vi "Write Pulse Recorder Configuration.vi"(8 "error in (no error)":errorcluster, 10 "Configuration":T1={"Pre-trigger duration"=0.01, "Post-trigger duration"=0.1, "Rate"=1000000.0, "Ranges"=[10.0], "Re-name channels"=[], "Active channels"="0:1", "External clock"=FALSE} {"Rate" format="%#_8pHz"; "Post-trigger duration" format="%#_6ps"; "Pre-trigger duration" format="%#_6ps"; "Ranges" format="%#_6pV"}, 11 "RP Delayed in":refnum<class "RP Level.lvclass">) -> (0 "error out":errorcluster, 3 "RP Delayed out":refnum<class "RP Level.lvclass">)   [LabVIEW 2016, in "RP Level.lvclass"]
uses:
  RP Level.lvclass
  NHMFL_Core/Libraries/Instruments/Pulse Driver/Pusle Driver Configuration.ctl
  NHMFL_Core/Libraries/Red Pitaya/RP Level Configuration.ctl
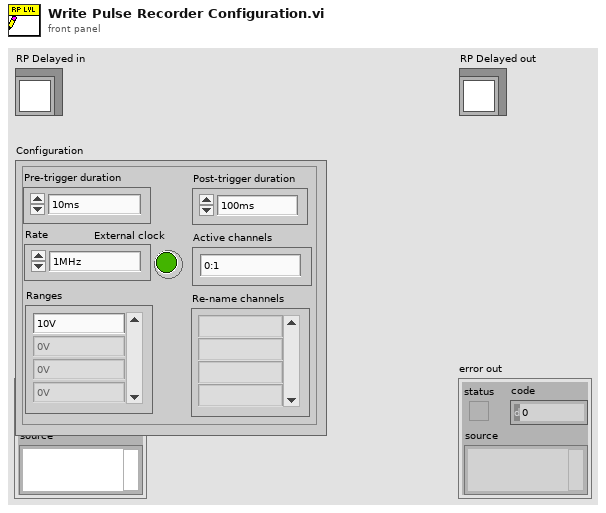
[diagram p1: front panel]
types:
  T1 = typedef "Pusle Driver Configuration.ctl" = cluster{"Pre-trigger duration":dbl, "Post-trigger duration":dbl, "Rate":dbl, "Ranges":dbl[], "Re-name channels":string[], "Active channels":string, "External clock":bool}
  T2 = typedef "RP Level Configuration.ctl" = cluster{"Pre-trigger duration":dbl, "Post-trigger duration":dbl, "Rate":dbl, "Ranges":dbl[], "Re-name channels":string[], "Active channels":string, "External clock":bool, "Output delay":dbl, "Raising edge ":bool, "Trigger level":dbl}
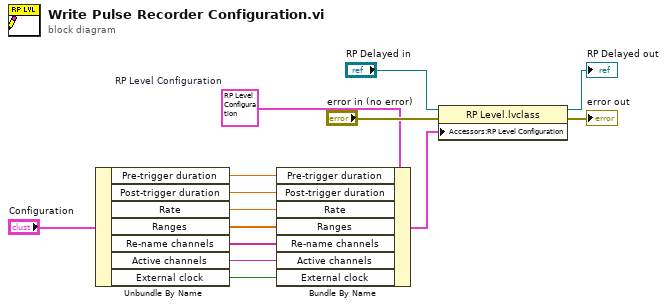
[diagram p0: block diagram]
diagram:
  w3 = T2 {"Pre-trigger duration"=0.01, "Post-trigger duration"=0.1, "Rate"=1000000.0, "Ranges"=[10.0], "Re-name channels"=[], "Active channels"="0:1", "External clock"=FALSE, "Output delay"=0.1, "Raising edge "=FALSE, "Trigger level"=0.001}  # RP Level Configuration
  n1 = Unbundle By Name("Configuration") -> ("Pre-trigger duration"=w4:dbl, "Post-trigger duration"=w5:dbl, "Rate"=w6:dbl, "Ranges"=w7:dbl[], "Re-name channels"=w8:string[], "Active channels"=w9:string, "External clock"=w10:bool)
  n2 = Bundle By Name(cluster=w3, "Pre-trigger duration"=w4, "Post-trigger duration"=w5, "Rate"=w6, "Ranges"=w7, "Re-name channels"=w8, "Active channels"=w9, "External clock"=w10) -> (w1:T2)
  n3 = property class="RP Level.lvclass"(reference="RP Delayed in", error in="error in (no error)", "Accessors:RP Level Configuration"=w1) -> (reference out=→"RP Delayed out":refnum<class "RP Level.lvclass">, error out=→"error out":errorcluster)
